vi "FdxCmdTxSAPBlockWriteCvi.vi"(8 "error in":errorcluster, 9 "SapBlockWriteIn":T2, 11 "InstrumentHandle":u32) -> (0 "error out":errorcluster, 1 "SapBlockWriteOut":T1, 3 "InstrumentHandle":u32)   [LabVIEW 2020, in "AIM664LV.lvlib"]
doc: "This function is used to write a pure message to one or more SAP ports. If the data size is not applicable for the data size associated to this port this function will return an error.\nThis function can be used if the transmitter is running or not running."
uses:
  AIM664LV.lvlib
  AFDX_LibraryAdmin/FdxGlobalDllPath.vi
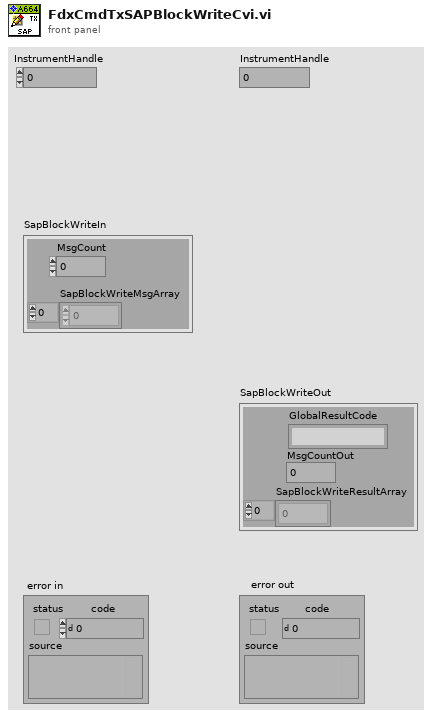
[diagram p1: front panel]
types:
  T1 = cluster{"GlobalResultCode":string, "MsgCountOut":u32, "SapBlockWriteResultArray":u8[]}
  T2 = cluster{"MsgCount":u32, "SapBlockWriteMsgArray":u8[]}
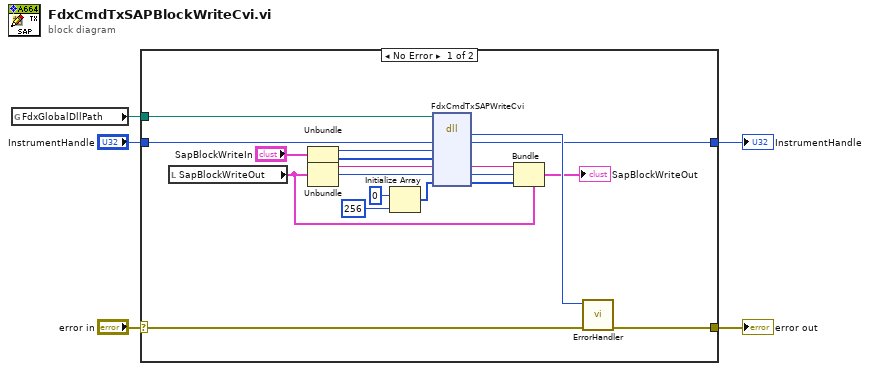
[diagram p0: block diagram]
diagram:
  n1 = global read "FdxGlobalDllPath.vi" "FdxGlobalDllPath"() -> (w3:path)
  n2 = case shown="No Error" "error in" {
    selector: "error in" -> [w23 w26]
    tunnel: [w24 w26] -> w5
    tunnel: w3 -> [w8 _]
    tunnel: "InstrumentHandle" -> [w7 w25]
    tunnel: [w6 w25] -> w1
    frame No Error {
      n3 = local read "SapBlockWriteOut"() -> (w11:T1)
      n4 = Unbundle("SapBlockWriteIn") -> ("MsgCount"=w18:u32, "SapBlockWriteMsgArray"=w13:u8[])
      n5 = Unbundle(w11) -> ("GlobalResultCode"=w9:string, "MsgCountOut"=w10:u32)  [unwired: 1 out]
      n6 = Initialize Array(u8 0 ("element"), 256 ("dimension size")) -> (w14:u8[])
      n7 = dll-call lib="aim_fdx.19.dll" fn="FdxCmdTxSAPWriteCvi"(path in=w8, "InstrumentHandle"=w7, "MsgCount"=w18, "SapBlockWriteMsgArray"=w13, "GlobalResultCode"=w9, "MsgCountOut"=w10, "SapBlockWriteResultArray"=w14) -> ("status"=w22:i32, "InstrumentHandle"=w6:u32, "GlobalResultCode"=w20:string, "MsgCountOut"=w19:u32, "SapBlockWriteResultArray"=w12:u8[])  [unwired: 4 in, 2 out]
      n8 = Bundle(cluster=w11, "GlobalResultCode"=w20, "MsgCountOut"=w19, "SapBlockWriteResultArray"=w12) -> (→"SapBlockWriteOut":T1)
      n9 = call "ErrorHandler.vi"("error in"=w23, "AIM Error"=w22) -> ("error out"=w24:errorcluster)  [unwired: 9 in]
    }
    frame Error {
    }
  }
  "error out" <- w5
  "InstrumentHandle" <- w1
